vi "Telescope Home Focus.vi"(8 "error in (no error)":errorcluster, 11 "Telescope Simulator in":refnum<class "Telescope Simulator.lvclass">) -> (0 "error out":errorcluster, 3 "Telescope Simulator out":refnum<class "Telescope Simulator.lvclass">)   [LabVIEW 2024, in "Telescope Simulator.lvclass"]
uses:
  Telescope Simulator.lvclass
  Telescope enum Status.ctl
  Telescope Simulator.lvclass/Telescope Simulator.ctl
  Telescope.lvclass
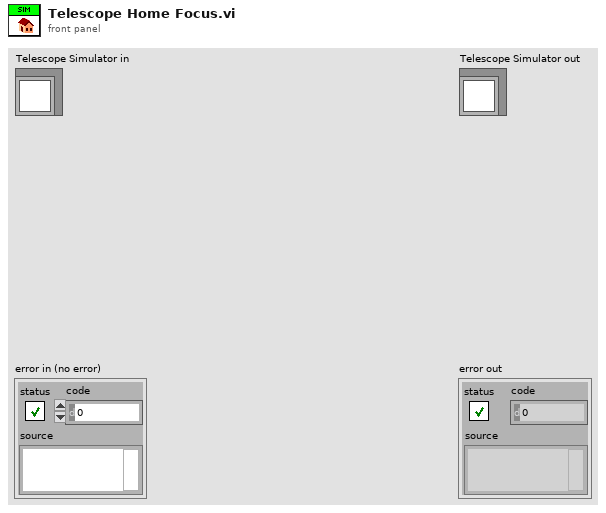
[diagram p1: front panel]
types:
  T1 = typedef "Telescope.lvclass/Telescope enum Status.ctl" = enum16{"Initializing", "Ready", "Moving", "Focusing", "Error"}
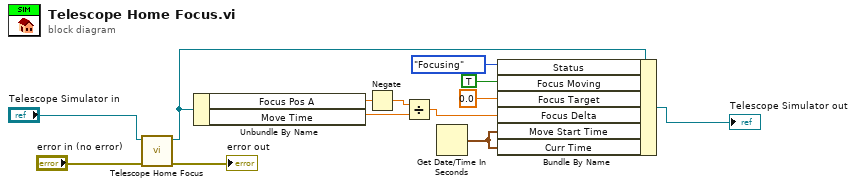
[diagram p0: block diagram]
diagram:
  n1 = call-parent "Telescope Home Focus.vi"("error in (no error)"="error in (no error)", "Telescope in"="Telescope Simulator in") -> ("error out"=→"error out":errorcluster, "Telescope out"=w9:refnum<class "Telescope Simulator.lvclass">)  [unwired: 8 in]
  n2 = Unbundle By Name(w9) -> ("Focus Pos A"=w11:dbl, "Move Time"=w10:dbl)
  n3 = Negate(x=w11) -> (-x=w1:dbl)
  n4 = Divide(x=w1, y=w10) -> (x/y=w8:dbl)
  n5 = Get Date/Time In Seconds() -> (seconds since 1Jan1904=w5:timestamp)
  n6 = Bundle By Name(cluster=w9, "Status"=Telescope_enum_Status."Focusing" ("Telescope Status.Status"), "Focus Moving"=TRUE ("Focus.Focus Moving"), "Focus Target"=0.0 ("Focus.Focus Target"), "Focus Delta"=w8, "Move Start Time"=w5, "Curr Time"=w5) -> (→"Telescope Simulator out":refnum<class "Telescope Simulator.lvclass">)
